vi "Write Width (us).vi"(8 "error in (no error)":errorcluster, 10 "Width (us)":string, 11 "Pulse Train in":refnum<class "Pulse Train.lvclass">) -> (0 "error out":errorcluster, 3 "Pulse Train out":refnum<class "Pulse Train.lvclass">)   [LabVIEW 2020, in "Pulse Train.lvclass"]
uses:
  Pulse Train.lvclass
  Pulse Train.lvclass/Pulse Train.ctl
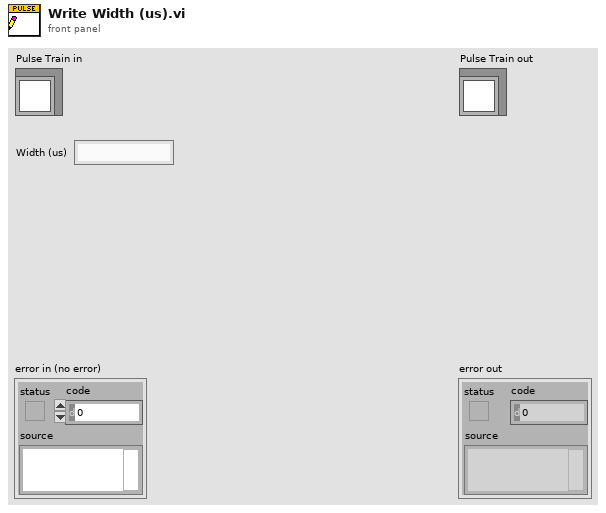
[diagram p1: front panel]
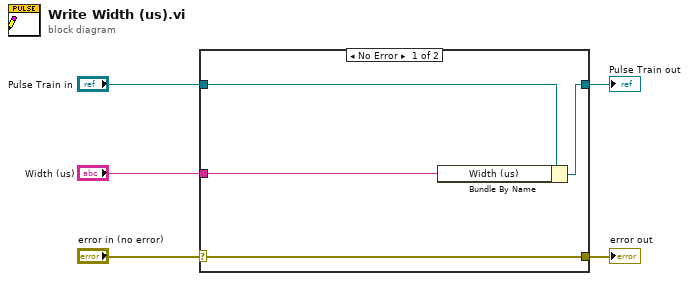
[diagram p0: block diagram]
diagram:
  n1 = case shown="No Error" "error in (no error)" {
    selector: "error in (no error)" -> [w9 w10]
    tunnel: [w9 w10] -> w4
    tunnel: [w7 w11] -> w2
    tunnel: "Pulse Train in" -> [w8 w11]
    tunnel: "Width (us)" -> [w6 _]
    frame No Error {
      n2 = Bundle By Name(cluster=w8, "Width (us)"=w6) -> (w7:refnum<class "Pulse Train.lvclass">)
    }
    frame Error {
    }
  }
  "error out" <- w4
  "Pulse Train out" <- w2
